vi "Read Tx Duration.vi"(8 "error in (no error)":errorcluster, 11 "Framework Performance in":refnum<class "Performance.lvclass">) -> (0 "error out":errorcluster, 2 "tx duration":u32 format="%d us", 3 "Framework Performance out":refnum<class "Performance.lvclass">)   [LabVIEW 2017, in "DSF Core.lvlib" / "Performance.lvclass"]
uses:
  Performance.lvclass
  Performance.lvclass/Performance.ctl
  Timing Status/Timing Status Size.vi
  Timing Status/Timing Status.lvclass
  C:/Git/DSF/LabVIEW-Memory/Source/Classes/Pointer/Pointer.lvclass
  LabVIEW-Memory/Source/Classes/Pointer/Get Address.vi
  LabVIEW-Memory/Source/Classes/Pointer/Check Size (0D).vi
  LabVIEW-Memory/Source/Classes/Pointer/Check Null Pointer.vi
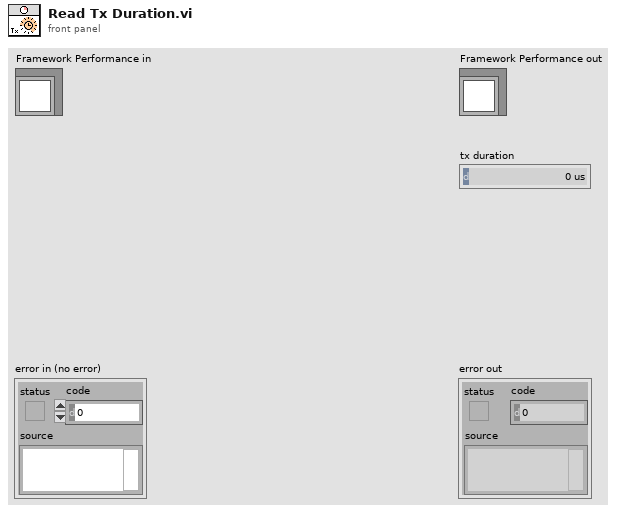
[diagram p1: front panel]
types:
  T1 = typedef "DSF Core.lvlib/Timing Status.lvclass/Timing Status Data.ctl" = cluster{"rx start time":u32, "rx end time":u32, "tx start time":u32, "tx end time":u32, "cycle start time":u32, "cycle end time":u32, "prev start time":u32}
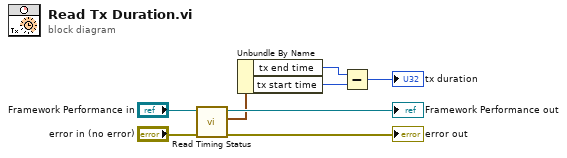
[diagram p0: block diagram]
diagram:
  n1 = call "Read Timing Status.vi"("error in (no error)"="error in (no error)", "Framework Performance in"="Framework Performance in") -> ("error out"=→"error out":errorcluster, "timing status"=w1:T1, "Framework Performance out"=→"Framework Performance out":refnum<class "Performance.lvclass">)  [unwired: 7 in]
  n2 = Unbundle By Name(w1) -> ("tx end time"=w8:u32, "tx start time"=w7:u32)
  n3 = Subtract(x=w8, y=w7) -> (x-y=→"tx duration":u32)
